vi "testCallParentTransceiverInterface.vi"(8 "error in (no error)":errorcluster, 11 "TestCase in":refnum<class "MockTransceiverTestCases.lvclass">) -> (0 "error out":errorcluster, 3 "TestCase out":refnum<class "MockTransceiverTestCases.lvclass">)   [LabVIEW 2017, in "MockTransceiverTestCases.lvclass"]
uses:
  MockTransceiverTestCases.lvclass
  Configuration/Public/Controls/DSF Engine Transfer Group Configuration.ctl
  Configuration/Public/Controls/DSF Direction.ctl
  Configuration/Public/Controls/DSF Timing Info.ctl
  Configuration/Public/Controls/DSF Engine Transfer Configuration.ctl
  Configuration/Public/Controls/DSF Byte Order.ctl
  Configuration/Public/Controls/DSF Engine Channel Configuration.ctl
  Configuration/Public/Controls/DSF Data Type.ctl
  Configuration/Public/Controls/DSF Settings Info.ctl
  Engine/Classes/Transceiver/Transceiver.lvclass
  Engine/Classes/Transfer Group/Transfer Group.lvclass
  <vilib>/addons/_JKI Toolkits/VI Tester/TestCase.llb/TestCase.lvclass
  DSF Core.lvlib
  C:/Program Files (x86)/National Instruments/LabVIEW 2017/vi.lib/addons/_JKI Toolkits/VI Tester/TestCase.llb/TestCase.lvclass
panel:
  in  "Transfer Groups Configurations":T1[](array[typedef]) {"Transfers"."channel configurations"."buffer offset" format="%d bytes"}
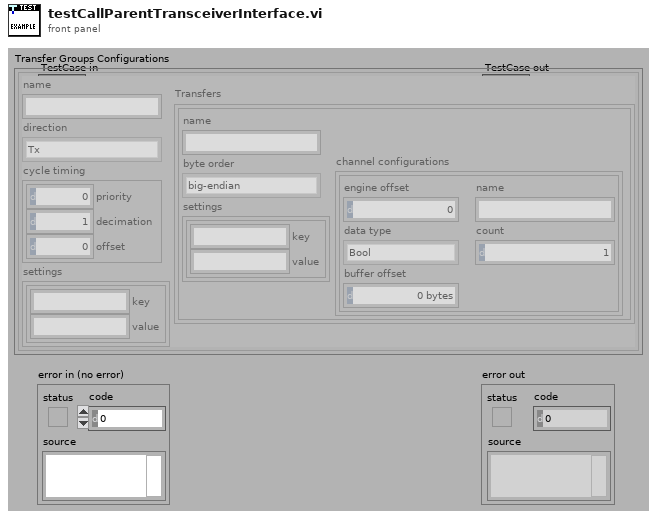
[diagram p1: front panel]
types:
  T1 = typedef "DSF Core.lvlib/DSF Engine Transfer Group Configuration.ctl" = cluster{"name":string, "direction":T2, "cycle timing":T3, "Transfers":T4[], "settings":T8}
  T2 = typedef "DSF Core.lvlib/DSF Direction.ctl" = enum8{"Tx", "Rx"}
  T3 = typedef "DSF Core.lvlib/DSF Timing Info.ctl" = cluster{"priority":u64, "decimation":u64, "offset":u64}
  T4 = typedef "DSF Core.lvlib/DSF Engine Transfer Configuration.ctl" = cluster{"name":string, "byte order":T5, "channel configurations":T6[], "settings":T8}
  T5 = typedef "DSF Core.lvlib/DSF Byte Order.ctl" = enum8{"big-endian", "little-endian"}
  T6 = typedef "DSF Core.lvlib/DSF Engine Channel Configuration.ctl" = cluster{"engine offset":u64, "name":string, "data type":T7, "count":u64, "buffer offset":u64}
  T7 = typedef "DSF Core.lvlib/DSF Data Type.ctl" = enum8{"Bool", "SGL", "DBL", "I8", "I16", "I32", "I64", "U8", "U16", "U32", "U64"}
  T8 = typedef "DSF Core.lvlib/DSF Settings Info.ctl" = cluster{"key":string, "value":string}[]
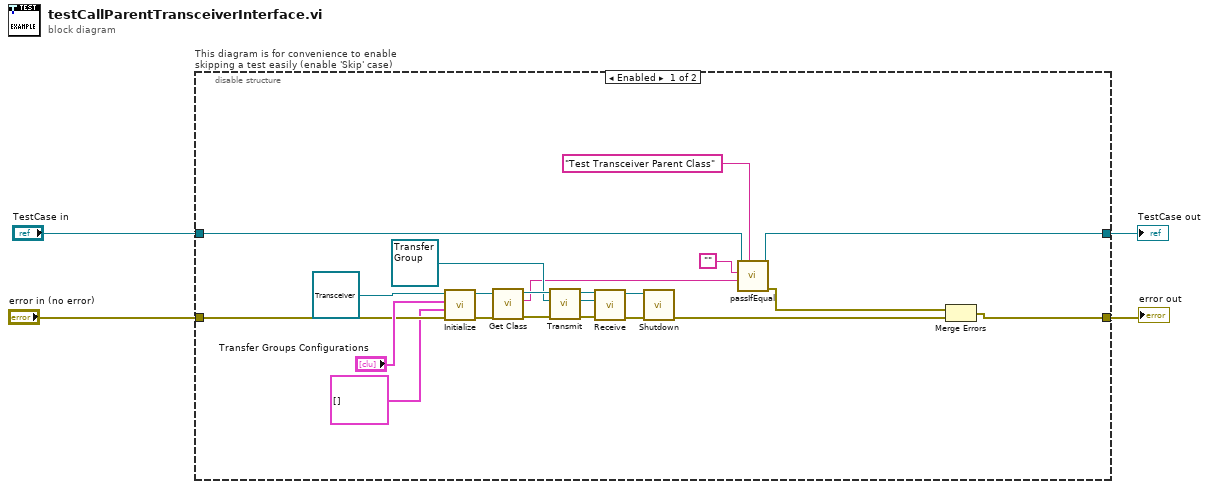
[diagram p0: block diagram]
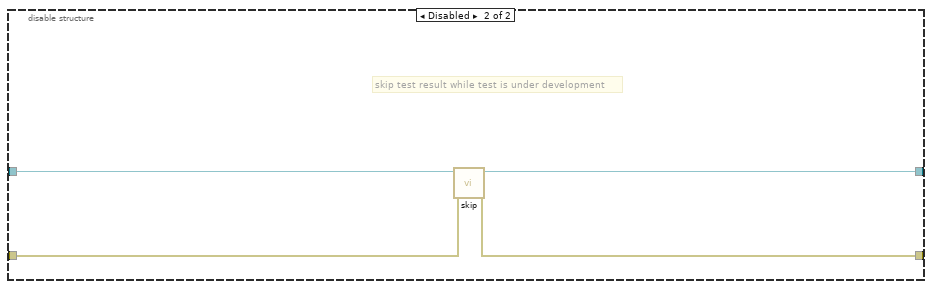
[diagram p2: hidden frame]
diagram:
  n1 = disable-structure "This diagram is for convenience to enable skipping a test easily (enable 'Skip' case)" shown="Enabled" {
    disable-tunnel: "TestCase in" -> [w26 w30]
    disable-tunnel: [w25 w28] -> w1
    disable-tunnel: [w20 w29] -> w3
    disable-tunnel: "error in (no error)" -> [w22 w27]
    frame Enabled {
      n2 = call-dynamic "Initialize.vi"("error in (no error)"=w22, "transceiver settings"=T8 [], "Transfer Groups Configurations"="Transfer Groups Configurations", "Transceiver in"=refnum<class "Transceiver.lvclass"> refnum) -> ("error out"=w19:errorcluster, "Transceiver out"=w18:refnum<class "Transceiver.lvclass">)  [unwired: 6 in]
      n3 = call-dynamic "Get Class.vi"("error in (no error)"=w19, "Transceiver in"=w18) -> ("error out"=w17:errorcluster, "class"=w6:string, "Transceiver out"=w16:refnum<class "Transceiver.lvclass">)  [unwired: 7 in]
      n4 = call-dynamic "Transmit.vi"("error in (no error)"=w17, "Transfer Group in"=refnum<class "Transfer Group.lvclass"> refnum, "Transceiver in"=w16) -> ("error out"=w15:errorcluster, "Transfer Group out"=w14:refnum<class "Transfer Group.lvclass">, "Transceiver out"=w13:refnum<class "Transceiver.lvclass">)  [unwired: 6 in]
      n5 = call-dynamic "Receive.vi"("error in (no error)"=w15, "Transfer Group in"=w14, "Transceiver in"=w13) -> ("error out"=w12:errorcluster, "Transceiver out"=w10:refnum<class "Transceiver.lvclass">)  [unwired: 6 in, 1 out]
      n6 = call-dynamic "Shutdown.vi"("error in (no error)"=w12, "Transceiver in"=w10) -> ("error out"=w11:errorcluster)  [unwired: 8 in, 1 out]
      n7 = call-dynamic "passIfEqual.vi"("custom report message (\"\")"="Test Transceiver Parent Class" ("custom report message (\"\")"), "y"=w6, "x"="", "TestCase in"=w26) -> ("error out"=w21:errorcluster, "TestCase out"=w25:refnum<class "MockTransceiverTestCases.lvclass">)  [unwired: 6 in]
      n8 = Merge Errors(w21, w11) -> (w20:errorcluster)
    }
    frame Disabled {
      # "skip test result while test is under development"
      n9 = call <vilib>:"skip.vi"("error in (no error)"=w27, "TestCase in"=w30) -> ("error out"=w29:errorcluster, "TestCase out"=w28:refnum<class "MockTransceiverTestCases.lvclass">)  [unwired: 8 in]
    }
  }
  "error out" <- w3
  "TestCase out" <- w1
